vi "Trigger.vi"(8 "error in (no error)":errorcluster, 11 "VISA resource name":refnum<visa-resource-name>) -> (0 "error out":errorcluster, 3 "VISA resource name out":refnum<visa-resource-name>)   [LabVIEW 2016, in "Agilent 4263X.lvlib"]
doc: "This VI sends the :TRIG to the instrument.\n\n:TRIG causes the trigger to execute a measurement, reguardless of the trigger state."
uses:
  <instrlib>/Agilent 4263X/Agilent 4263X.lvlib
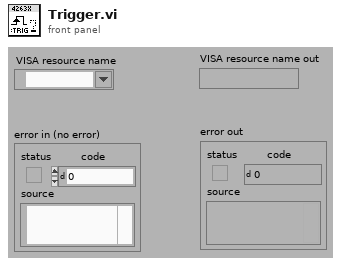
[diagram p1: front panel]
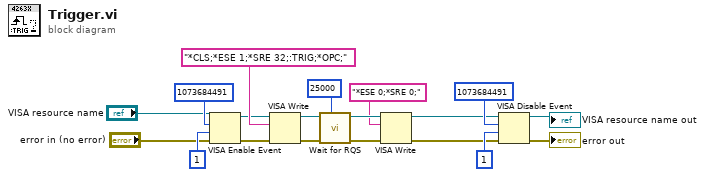
[diagram p0: block diagram]
diagram:
  n1 = VISA Enable Event(8:"error in (no error)", 9:u16 1, 10:u32 1073684491, 11:"VISA resource name") -> (0:w9:errorcluster, 3:w8:refnum<visa-resource-name>)
  n2 = VISA Write(VISA resource name=w8, write buffer="*CLS;*ESE 1;*SRE 32;:TRIG;*OPC;", error in (no error)=w9) -> (VISA resource name out=w19:refnum<visa-resource-name>, error out=w18:errorcluster)  [unwired: 1 out]
  n3 = call <vilib>:"Wait for RQS.VI"("timeout (25000 ms)"=u32 25000, "error in (no error)"=w18, "VISA resource name"=w19) -> ("error out"=w16:errorcluster, "VISA resource name out"=w17:refnum<visa-resource-name>)  [unwired: 6 in, 1 out]
  n4 = VISA Write(VISA resource name=w17, write buffer="*ESE 0;*SRE 0;", error in (no error)=w16) -> (VISA resource name out=w1:refnum<visa-resource-name>, error out=w4:errorcluster)  [unwired: 1 out]
  n5 = VISA Disable Event(8:w4, 9:u16 1, 10:u32 1073684491, 11:w1) -> (0:→"error out":errorcluster, 3:→"VISA resource name out":refnum<visa-resource-name>)
